vi "Изменение коэффициентов.vi"(0 "VISA Refnum in":refnum<visa-resource-name>, 1 "KP_ugol_z":dbl(slide) scale=0.0..100.0, 2 "KD_vel":dbl(slide) scale=0.0..0.3, 3 "KP_ugol_z_b":bool, 4 "KD_vel 2":bool, 5 "error in (no error)":errorcluster, 6 "KI_vel 2":bool, 7 "KI_ugla 2":bool, 8 "KP_ugla":dbl(slide) scale=0.0..500.0, 9 "KI_ugla":dbl(slide) scale=0.0..100.0, 10 "KP_ugla 2":bool, 11 "KP_vel 2":bool, 12 "KI_vel":dbl(slide) scale=0.0..100.0, 13 "KP_vel":dbl(slide) scale=0.0..500.0, 14 "KP_vel_z_b":bool, 15 "KP_vel_z":dbl(slide) scale=0.0..0.3, 16 "KD_vel_z_b":bool, 17 "KD_vel_z":dbl(slide) scale=0.0..100.0, 18 "KI_vel_z":dbl(slide) scale=0.0..100.0, 19 "KI_vel_z_b":bool) -> ()   [LabVIEW 2013]
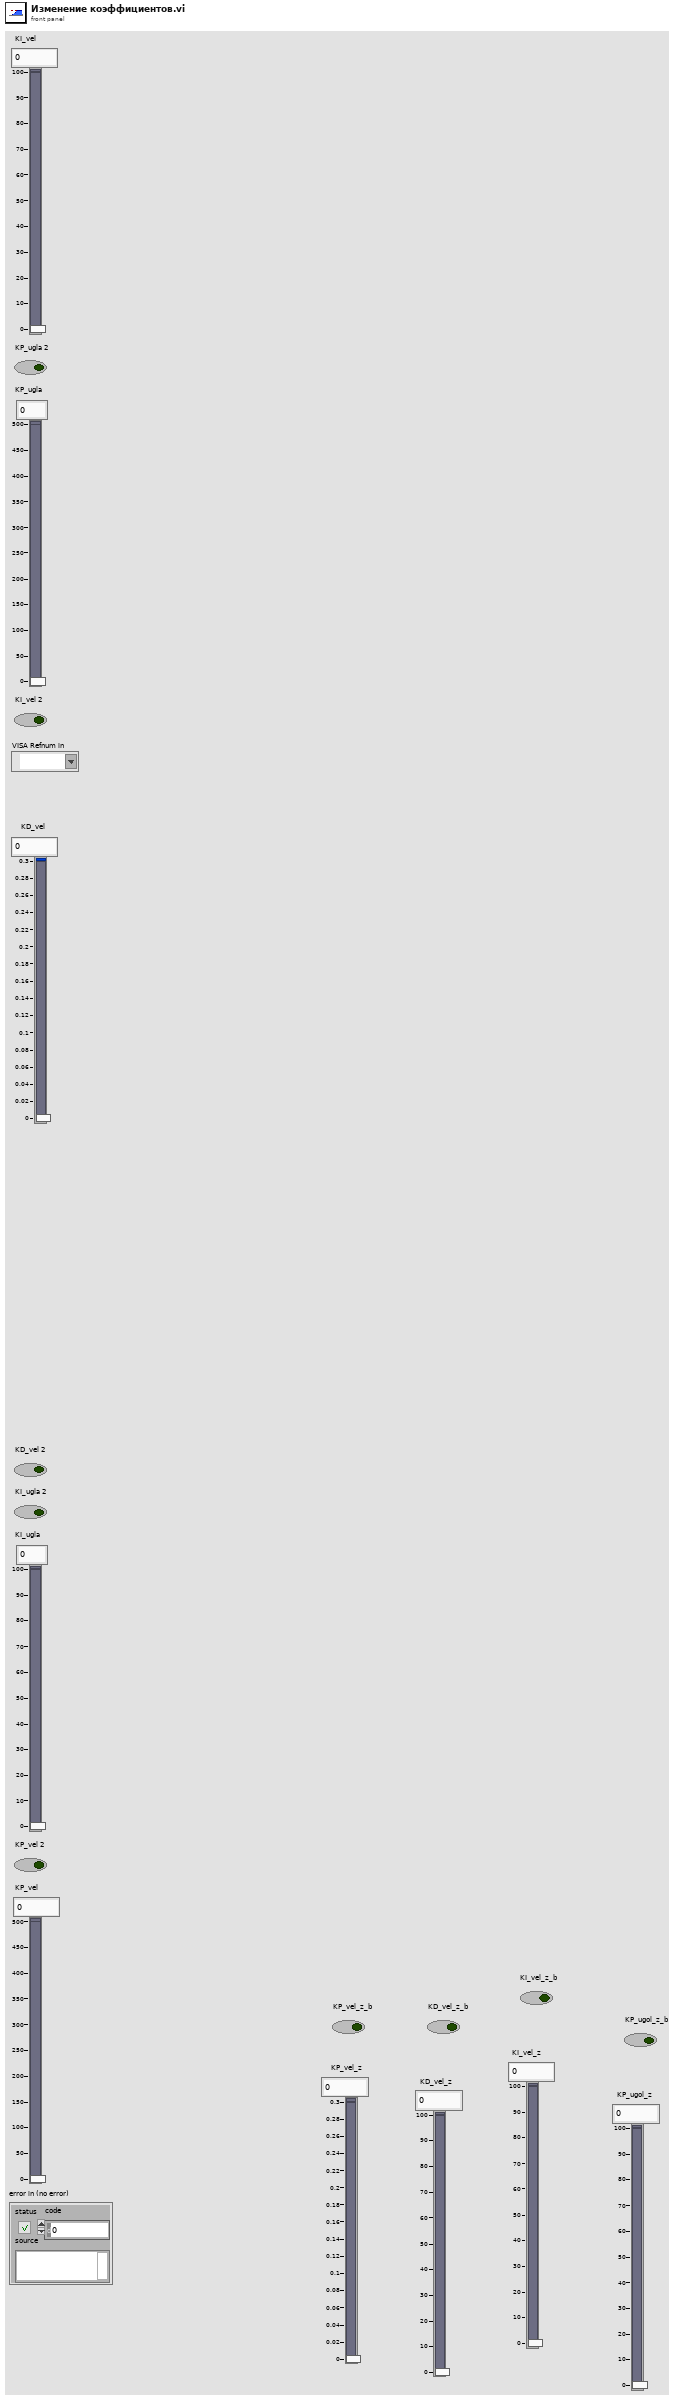
[diagram p1: front panel]
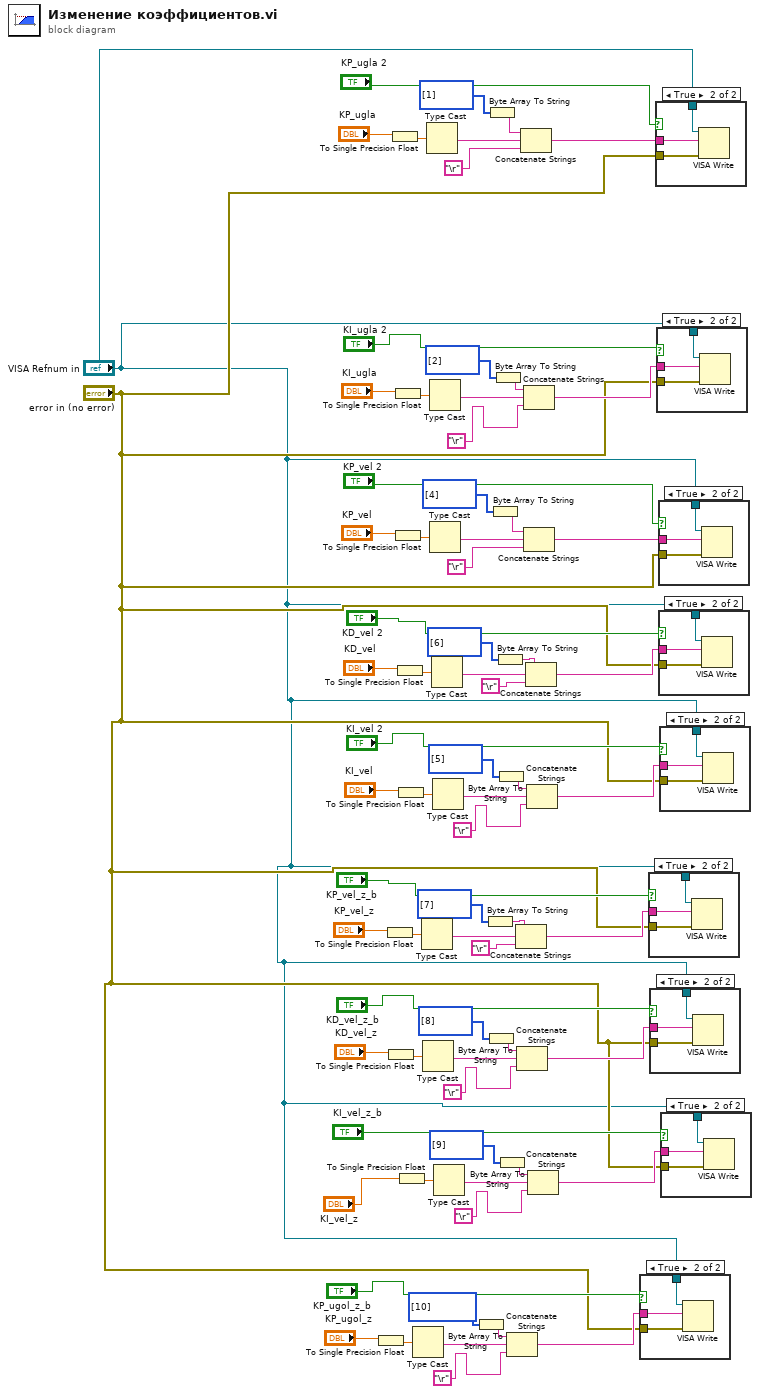
[diagram p0: block diagram]
diagram:
  n1 = To Single Precision Float(number="KP_ugol_z") -> (single precision float=w4:sgl)
  n2 = To Single Precision Float(number="KP_vel_z") -> (single precision float=w28:sgl)
  n3 = To Single Precision Float(number="KD_vel_z") -> (single precision float=w20:sgl)
  n4 = To Single Precision Float(number="KP_ugla") -> (single precision float=w36:sgl)
  n5 = To Single Precision Float(number="KI_ugla") -> (single precision float=w40:sgl)
  n6 = To Single Precision Float(number="KP_vel") -> (single precision float=w52:sgl)
  n7 = To Single Precision Float(number="KD_vel") -> (single precision float=w68:sgl)
  n8 = To Single Precision Float(number="KI_vel") -> (single precision float=w56:sgl)
  n9 = To Single Precision Float(number="KI_vel_z") -> (single precision float=w14:sgl)
  n10 = Type Cast(x=w4) -> (*(type *) &x=w3:string)  [unwired: 1 in]
  n11 = Type Cast(x=w28) -> (*(type *) &x=w27:string)  [unwired: 1 in]
  n12 = Type Cast(x=w20) -> (*(type *) &x=w19:string)  [unwired: 1 in]
  n13 = Type Cast(x=w36) -> (*(type *) &x=w35:string)  [unwired: 1 in]
  n14 = Type Cast(x=w40) -> (*(type *) &x=w39:string)  [unwired: 1 in]
  n15 = Type Cast(x=w52) -> (*(type *) &x=w51:string)  [unwired: 1 in]
  n16 = Type Cast(x=w68) -> (*(type *) &x=w67:string)  [unwired: 1 in]
  n17 = Type Cast(x=w56) -> (*(type *) &x=w55:string)  [unwired: 1 in]
  n18 = Type Cast(x=w14) -> (*(type *) &x=w13:string)  [unwired: 1 in]
  n19 = Byte Array To String(unsigned byte array=u8[] [10]) -> (string=w10:string)
  n20 = Byte Array To String(unsigned byte array=u8[] [7]) -> (string=w34:string)
  n21 = Byte Array To String(unsigned byte array=u8[] [8]) -> (string=w26:string)
  n22 = Byte Array To String(unsigned byte array=u8[] [1]) -> (string=w47:string)
  n23 = Byte Array To String(unsigned byte array=u8[] [4]) -> (string=w63:string)
  n24 = Byte Array To String(unsigned byte array=u8[] [2]) -> (string=w50:string)
  n25 = Byte Array To String(unsigned byte array=u8[] [6]) -> (string=w74:string)
  n26 = Byte Array To String(unsigned byte array=u8[] [5]) -> (string=w66:string)
  n27 = Byte Array To String(unsigned byte array=u8[] [9]) -> (string=w18:string)
  n28 = Concatenate Strings(w10, w3, "\r") -> (w7:string)
  n29 = Concatenate Strings(w34, w27, "\r") -> (w31:string)
  n30 = Concatenate Strings(w26, w19, "\r") -> (w23:string)
  n31 = Concatenate Strings(w47, w35, "\r") -> (w43:string)
  n32 = Concatenate Strings(w50, w39, "\r") -> (w44:string)
  n33 = Concatenate Strings(w63, w51, "\r") -> (w59:string)
  n34 = Concatenate Strings(w74, w67, "\r") -> (w71:string)
  n35 = Concatenate Strings(w66, w55, "\r") -> (w60:string)
  n36 = Concatenate Strings(w18, w13, "\r") -> (w16:string)
  n37 = case shown="True" "KP_ugol_z_b" {
    tunnel: w7 -> [_ w77]
    tunnel: "VISA Refnum in" -> [_ w76]
    tunnel: "error in (no error)" -> [_ w75]
    frame False {
    }
    frame True {
      n38 = VISA Write(VISA resource name=w76, write buffer=w77, error in (no error)=w75) -> ()  [unwired: 3 out]
    }
  }
  n39 = case shown="True" "KP_vel_z_b" {
    tunnel: w31 -> [_ w80]
    tunnel: "VISA Refnum in" -> [_ w79]
    tunnel: "error in (no error)" -> [_ w78]
    frame False {
    }
    frame True {
      n40 = VISA Write(VISA resource name=w79, write buffer=w80, error in (no error)=w78) -> ()  [unwired: 3 out]
    }
  }
  n41 = case shown="True" "KD_vel_z_b" {
    tunnel: w23 -> [_ w83]
    tunnel: "VISA Refnum in" -> [_ w82]
    tunnel: "error in (no error)" -> [_ w81]
    frame False {
    }
    frame True {
      n42 = VISA Write(VISA resource name=w82, write buffer=w83, error in (no error)=w81) -> ()  [unwired: 3 out]
    }
  }
  n43 = case shown="True" "KP_ugla 2" {
    tunnel: w43 -> [_ w86]
    tunnel: "VISA Refnum in" -> [_ w85]
    tunnel: "error in (no error)" -> [_ w84]
    frame False {
    }
    frame True {
      n44 = VISA Write(VISA resource name=w85, write buffer=w86, error in (no error)=w84) -> ()  [unwired: 3 out]
    }
  }
  n45 = case shown="True" "KI_ugla 2" {
    tunnel: w44 -> [_ w89]
    tunnel: "VISA Refnum in" -> [_ w88]
    tunnel: "error in (no error)" -> [_ w87]
    frame False {
    }
    frame True {
      n46 = VISA Write(VISA resource name=w88, write buffer=w89, error in (no error)=w87) -> ()  [unwired: 3 out]
    }
  }
  n47 = case shown="True" "KP_vel 2" {
    tunnel: w59 -> [_ w92]
    tunnel: "VISA Refnum in" -> [_ w91]
    tunnel: "error in (no error)" -> [_ w90]
    frame False {
    }
    frame True {
      n48 = VISA Write(VISA resource name=w91, write buffer=w92, error in (no error)=w90) -> ()  [unwired: 3 out]
    }
  }
  n49 = case shown="True" "KD_vel 2" {
    tunnel: w71 -> [_ w95]
    tunnel: "VISA Refnum in" -> [_ w94]
    tunnel: "error in (no error)" -> [_ w93]
    frame False {
    }
    frame True {
      n50 = VISA Write(VISA resource name=w94, write buffer=w95, error in (no error)=w93) -> ()  [unwired: 3 out]
    }
  }
  n51 = case shown="True" "KI_vel 2" {
    tunnel: w60 -> [_ w98]
    tunnel: "VISA Refnum in" -> [_ w97]
    tunnel: "error in (no error)" -> [_ w96]
    frame False {
    }
    frame True {
      n52 = VISA Write(VISA resource name=w97, write buffer=w98, error in (no error)=w96) -> ()  [unwired: 3 out]
    }
  }
  n53 = case shown="True" "KI_vel_z_b" {
    tunnel: w16 -> [_ w101]
    tunnel: "VISA Refnum in" -> [_ w100]
    tunnel: "error in (no error)" -> [_ w99]
    frame False {
    }
    frame True {
      n54 = VISA Write(VISA resource name=w100, write buffer=w101, error in (no error)=w99) -> ()  [unwired: 3 out]
    }
  }
